vi "Write BallonTipText.vi"(8 "error in (no error)":errorcluster, 10 "BallonTipText":string, 11 "BalloonTip in":refnum<class "BalloonTip.lvclass">) -> (0 "error out":errorcluster, 3 "BalloonTip out":refnum<class "BalloonTip.lvclass">)   [LabVIEW 2016, in "BalloonTip.lvclass"]
uses:
  BalloonTip.lvclass
  BalloonTip.lvclass/BalloonTip.ctl
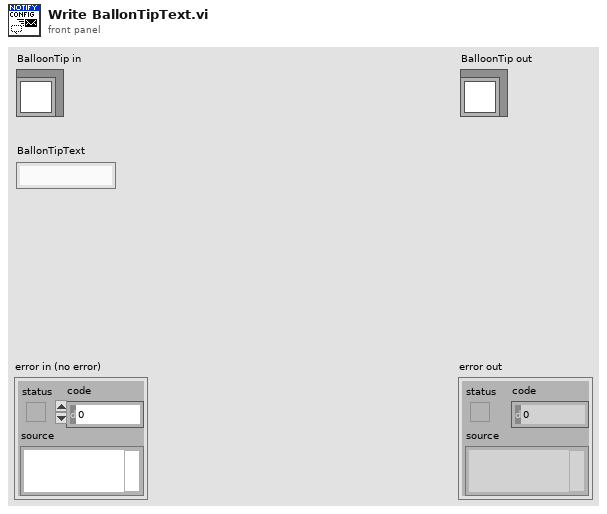
[diagram p1: front panel]
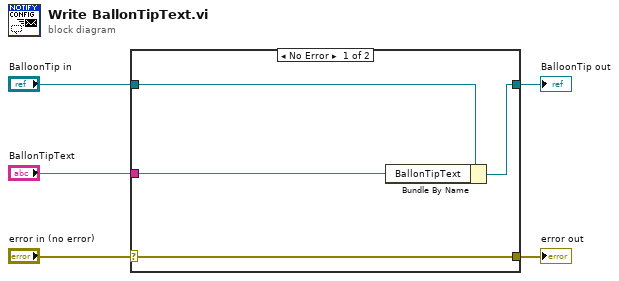
[diagram p0: block diagram]
diagram:
  n1 = case shown="No Error" "error in (no error)" {
    selector: "error in (no error)" -> [w9 w10]
    tunnel: [w9 w10] -> w4
    tunnel: [w7 w11] -> w2
    tunnel: "BalloonTip in" -> [w8 w11]
    tunnel: "BallonTipText" -> [w6 _]
    frame No Error {
      n2 = Bundle By Name(cluster=w8, "BallonTipText"=w6) -> (w7:refnum<class "BalloonTip.lvclass">)
    }
    frame Error {
    }
  }
  "error out" <- w4
  "BalloonTip out" <- w2
